vi "Copy Data from cRIO.vi"(6 "cRIO Address":string="192.168.1.x", 11 "Transferring Data to PC":refnum<vi>) -> (0 "error out":errorcluster)   [LabVIEW 2013]
doc: "Copies data from the default data directory on the specified cRIO (or RT target).\n\n\nVersion 1.0 - 02/13/2013\n\nPhaeron, Inc.\nwww.phaeron.com\ninfo@phaeron.com"
uses:
  <vilib>/FTP/NI_FTP.lvlib
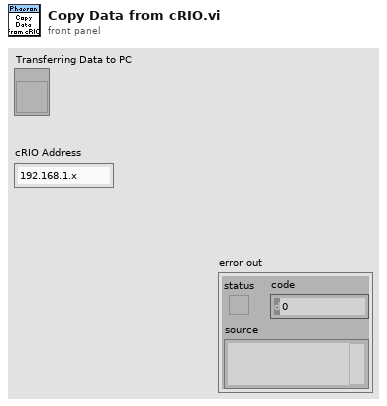
[diagram p1: front panel]
types:
  T1 = cluster{"remote path":string, "local path":path, "binary":bool}
  T2 = typedef "NI_FTP.lvlib/FTP Session.ctl" = refnum<k5>
  T3 = typedef "NI_FTP.lvlib/FTP File Info.ctl" = cluster{"type":enum16{"unknown", "file", "dir", "link"}, "permissions":string, "owner":string, "group":string, "size":i32, "date":string, "name":string, "link name":string}
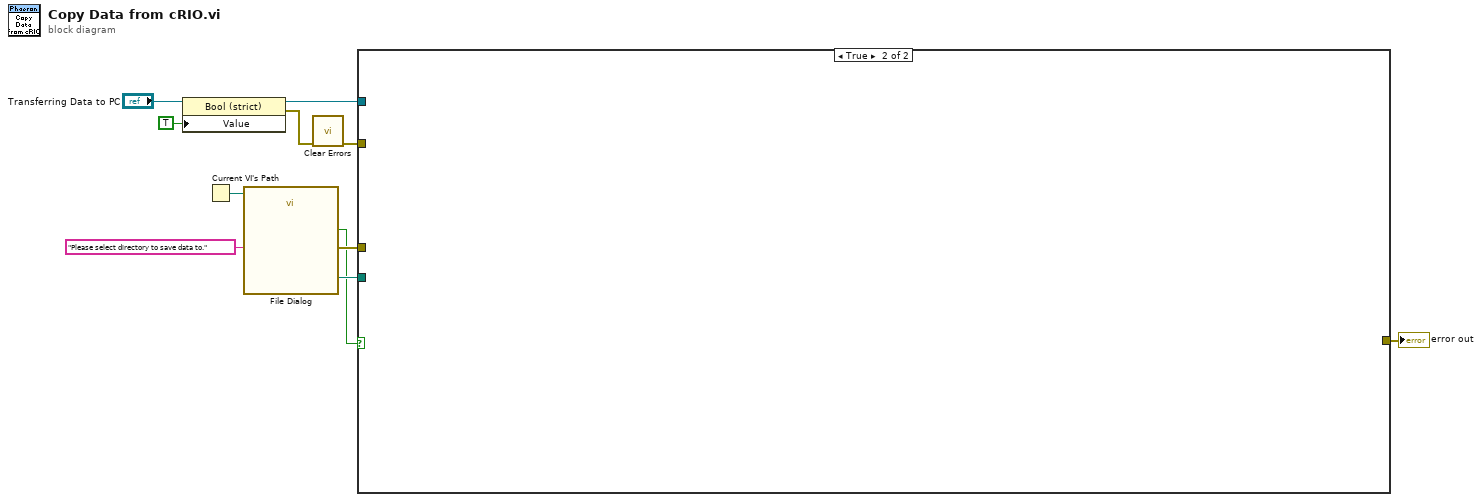
[diagram p0: block diagram]
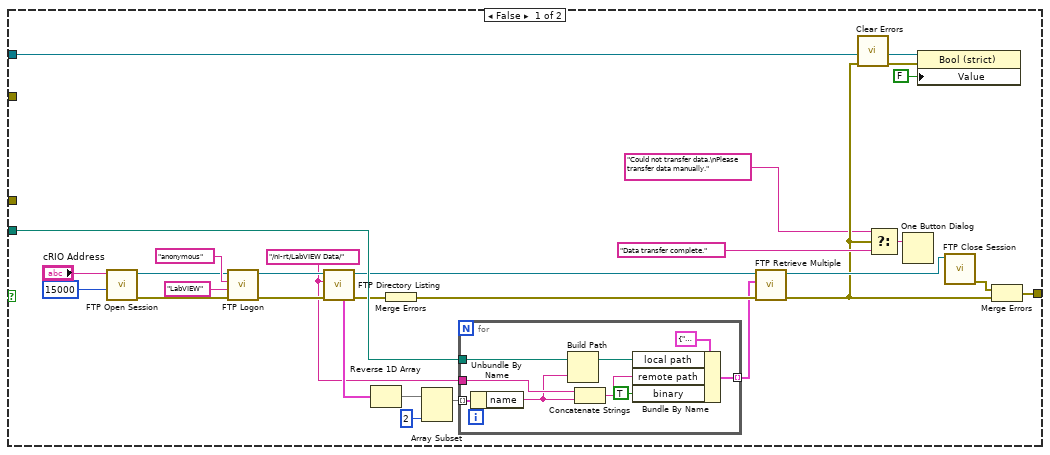
[diagram p2: hidden frame]
diagram:
  n1 = property class="Bool (strict)"(reference="Transferring Data to PC", "Value"=TRUE) -> (reference out=w3:refnum<vi>, error out=w2:errorcluster)  [unwired: 1 in]
  n2 = Current VI's Path() -> (path=w8:path)
  n3 = call "File Dialog"("start path"=w8, "prompt"="Please select directory to save data to.") -> ("selected path"=w9:path, "cancelled"=w6:bool, "error out"=w7:errorcluster)  [unwired: 10 in, 1 out]
  n4 = call <vilib>:"Clear Errors.vi"("error in (no error)"=w2) -> ("error out"=w1:errorcluster)  [unwired: 6 in]
  n5 = case shown="True" w6 {
    tunnel: w9 -> [w27 _]
    tunnel: [w23 _] -> w11
    tunnel: w7 -> [_ _]
    tunnel: w3 -> [w15 _]
    tunnel: w1 -> [_ _]
    frame False {
      w28 = "/ni-rt/LabVIEW Data/" ("directory path")
      n6 = call <vilib>:"FTP Open Session.vi"("timeout ms (60000)"=15000, "address"="cRIO Address") -> ("error out"=w30:errorcluster, "ftp session"=w31:T2)  [unwired: 6 in, 2 out]
      n7 = call <vilib>:"FTP Logon.vi"("error in (no error)"=w30, "password"="LabVIEW", "user"="anonymous", "ftp session"=w31) -> ("error out"=w33:errorcluster, "ftp session out"=w32:T2)  [unwired: 4 in, 2 out]
      n8 = call <vilib>:"FTP Directory Listing.vi"("error in (no error)"=w33, "directory path"=w28, "ftp session"=w32) -> ("error out"=w26:errorcluster, "ftp session out"=w25:T2, "dir list"=w36:T3[])  [unwired: 4 in, 2 out]
      n9 = Reverse 1D Array(array=w36) -> (reversed array=w37:T3[])
      n10 = Merge Errors(w26) -> (w21:errorcluster)
      n11 = Array Subset(array=w37, length=2) -> (w38:T3[])  [unwired: 1 in]
      n12 = for {
        tunnel: w38 -> [w48] mode=indexing
        tunnel: w28 -> [w47]
        tunnel: w27 -> [w44]
        tunnel: [w41] -> w20 mode=indexing
        n13 = Unbundle By Name(w48) -> ("name"=w42:string)
        n14 = Build Path(base path=w44, name or relative path=w42) -> (appended path=w43:path)
        n15 = Concatenate Strings(w47, w42) -> (w45:string)
        n16 = Bundle By Name(cluster=T1 {"remote path"="", "local path"=path "", "binary"=FALSE} ("transfer spec"), "local path"=w43, "remote path"=w45, "binary"=TRUE) -> (w41:T1)
      }
      n17 = call <vilib>:"FTP Retrieve Multiple.vi"("error in (no error)"=w21, "file specifications"=w20, "ftp session"=w25) -> ("error out"=w14:errorcluster, "ftp session out"=w24:T2)  [unwired: 5 in, 2 out]
      n18 = call <vilib>:"Clear Errors.vi"("error in (no error)"=w14) -> ("error out"=w16:errorcluster)  [unwired: 6 in]
      n19 = Select(t="Could not transfer data.\nPlease transfer data manually.", s=w14, f="Data transfer complete.") -> (s? t:f=w18:string)
      n20 = One Button Dialog(message=w18) -> ()  [unwired: 1 in, 1 out]
      n21 = property class="Bool (strict)"(reference=w15, error in=w16, "Value"=FALSE) -> ()  [unwired: 2 out]
      n22 = call <vilib>:"FTP Close Session.vi"("ftp session"=w24) -> ("error out"=w22:errorcluster)  [unwired: 7 in, 3 out]
      n23 = Merge Errors(w22, w14) -> (w23:errorcluster)
    }
    frame True {
    }
  }
  "error out" <- w11
